vi "Disable-Enable Button.vi"(8 "error in":errorcluster, 9 "Enabled?":bool, 11 "Data Loop Data in":T1) -> (0 "error out":errorcluster, 3 "Data Loop Data out":T1)   [LabVIEW 2018]
uses:
  Type Defs/Data Loop Data.ctl
  Support/Message Queue/Message Cluster.ctl
  Support/Message Queue/Message Queue.lvlib
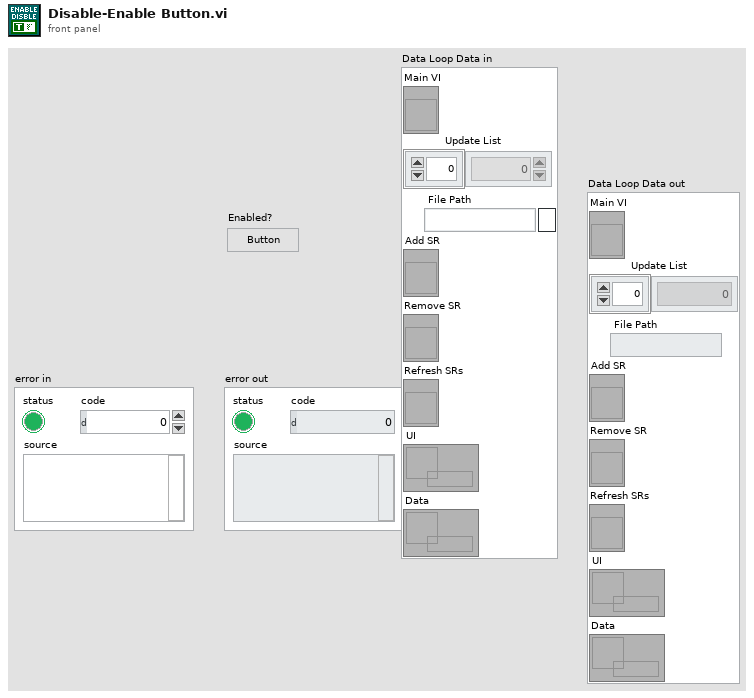
[diagram p1: front panel]
types:
  T1 = typedef "Data Loop Data.ctl" = cluster{"Main VI":refnum<vi>, "Update List":i32[], "File Path":path, "Add SR":refnum<vi>, "Remove SR":refnum<vi>, "Refresh SRs":refnum<vi>, "UI":refnum<queue>, "Data":refnum<queue>}
  T2 = enum8{"Enabled", "Disabled", "Disabled and Grayed Out"}
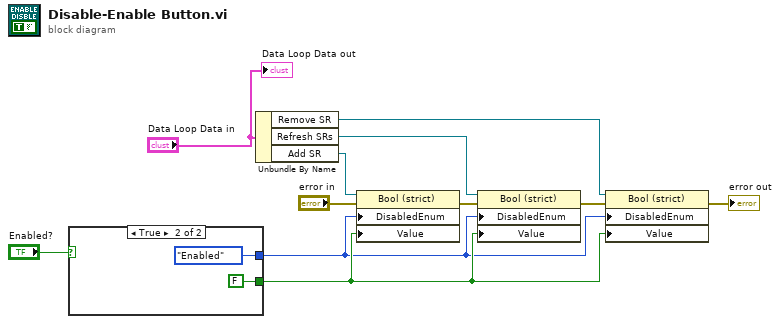
[diagram p0: block diagram]
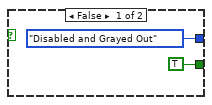
[diagram p2: hidden frame]
diagram:
  n1 = case shown="True" "Enabled?" {
    tunnel: [T2."Disabled and Grayed Out" ("Disabled") T2."Enabled" ("Disabled")] -> w1
    tunnel: [TRUE FALSE] -> w3
    frame False {
    }
    frame True {
    }
  }
  n2 = Unbundle By Name("Data Loop Data in") -> ("Remove SR"=w4:refnum<vi>, "Refresh SRs"=w7:refnum<vi>, "Add SR"=w8:refnum<vi>)
  n3 = property class="Bool (strict)"(reference=w8, error in="error in", "DisabledEnum"=w1, "Value"=w3) -> (error out=w11:errorcluster)  [unwired: 1 out]
  n4 = property class="Bool (strict)"(reference=w7, error in=w11, "DisabledEnum"=w1, "Value"=w3) -> (error out=w5:errorcluster)  [unwired: 1 out]
  n5 = property class="Bool (strict)"(reference=w4, error in=w5, "DisabledEnum"=w1, "Value"=w3) -> (error out=→"error out":errorcluster)  [unwired: 1 out]
  "Data Loop Data out" <- "Data Loop Data in"
